vi "CRC异或子VI.vi"(1 "输入":string) -> (0 "输出":string)   [LabVIEW 2013]
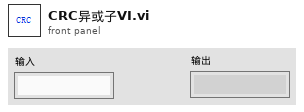
[diagram p1: front panel]
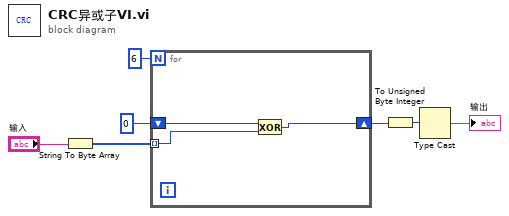
[diagram p0: block diagram]
diagram:
  n1 = String To Byte Array(string="输入") -> (unsigned byte array=w4:u8[])
  n2 = for {
    N: 6 -> [_]
    shift-right: [w8] -> w2
    shift-left: u8 0 -> [w10]
    tunnel: w4 -> [w9] mode=indexing
    n3 = Exclusive Or(1:w9, 2:w10) -> (0:w8:u8)
  }
  n4 = To Unsigned Byte Integer(number=w2) -> (unsigned 8bit integer=w1:u8)
  n5 = Type Cast(x=w1) -> (*(type *) &x=→"输出":string)  [unwired: 1 in]
